vi "Mixing Interface.vi"(10 "Owning VI":refnum<vi>, 11 "Shutdown Event":refnum<user-event>) -> ()   [LabVIEW 2020, in "User Interface.lvlib"]
doc: "Main control interface to Dataflow DJ. Also handles all keyboard shortcuts.\n\n<b>Execution System:</b> User Interface"
uses:
  User Interface.lvlib
  Custom Graphics/Slide.PlaybackPosition.ctl
  Custom Graphics/WaveformGraph.WaveformDisplay.ctl
  Custom Graphics/Button.Large.ctl
  Custom Graphics/LED.Red.16px.ctl
  <vilib>/Utility/miscctls.llb/LVCursorListTypeDef.ctl
  Packed Libraries/Audio Processing.lvlibp/Value Properties.ctl
  Packed Libraries/Messaging.lvlibp/Message Cluster.ctl
  Controls/Keyboard Shortcut.ctl
  Knob Fill.vi
  <vilib>/Utility/Data Type/Get Type Information.vi
  Packed Libraries/Messaging.lvlibp
  user32.dll
  Packed Libraries/Audio Processing.lvlibp
panel:
  in  "Transport.Record":T1
  in  "Mixer.Master":dbl(knob)=1.0 caption="MASTER" scale=0.0..1.0
  out "Mixer.Right.LevelIndicator":u8(slide) scale=0.0..20.0
  out "Mixer.Left.LevelIndicator":u8(slide) scale=0.0..20.0
  in  "Sample Pad.13.Trigger":T1
  in  "Sample Pad.14.Trigger":T1
  in  "Sample Pad.15.Trigger":T1
  in  "Sample Pad.16.Trigger":T1
  in  "Sample Pad.9.Trigger":T1
  in  "Sample Pad.10.Trigger":T1
  in  "Sample Pad.11.Trigger":T1
  in  "Sample Pad.12.Trigger":T1
  in  "Sample Pad.5.Trigger":T1
  in  "Sample Pad.6.Trigger":T1
  in  "Sample Pad.7.Trigger":T1
  in  "Sample Pad.8.Trigger":T1
  in  "Sample Pad.4.Trigger":T1
  in  "Sample Pad.3.Trigger":T1
  in  "Sample Pad.2.Trigger":T1
  in  "Sample Pad.1.Trigger":T1
  in  "Transport.Play":T1
  in  "Deck8.PlaybackPosition":T2 scale=0.0..15965568.0
  out "Deck8.Waveform":T3
  out "Deck8.Title":string
  in  "Channel8.Level":dbl(slide)=1.0 scale=0.0..1.0
  in  "EffectUnit8.Effect1.Enable":T4
  out "Channel8.LevelIndicator":u8(slide) scale=0.0..20.0
  in  "EffectUnit8.Effect1":u16(ring)=2 items=["CRUSHER", "ECHO", "FLANGER"]
  in  "Channel8.Gain":dbl(knob)=1.0 caption="GAIN" scale=0.0..2.0
  in  "Channel8.EQFilter":dbl(knob) caption="FILTER" scale=-1.025..1.025
  in  "EffectUnit8.Effect1.Value1":dbl(knob) caption="AMOUNT" scale=0.0..1.0
  in  "EffectUnit8.Effect1.Value2":dbl(knob) caption="SPEED" scale=0.0..0.1
  in  "Deck8.Reverse":T1
  in  "Deck8.Brake":T1
  in  "Deck8.Play":T1
  in  "Deck7.PlaybackPosition":T2 scale=0.0..15965568.0
  out "Deck7.Waveform":T3
  out "Deck7.Title":string
  in  "Channel7.Level":dbl(slide)=1.0 scale=0.0..1.0
  in  "EffectUnit7.Effect1.Enable":T4
  out "Channel7.LevelIndicator":u8(slide) scale=0.0..20.0
  in  "EffectUnit7.Effect1":u16(ring)=2 items=["CRUSHER", "ECHO", "FLANGER"]
  in  "Channel7.Gain":dbl(knob)=1.0 caption="GAIN" scale=0.0..2.0
  in  "Channel7.EQFilter":dbl(knob) caption="FILTER" scale=-1.025..1.025
  in  "EffectUnit7.Effect1.Value1":dbl(knob) caption="AMOUNT" scale=0.0..1.0
  in  "EffectUnit7.Effect1.Value2":dbl(knob) caption="SPEED" scale=0.0..0.1
  in  "Deck7.Reverse":T1
  in  "Deck7.Brake":T1
  in  "Deck7.Play":T1
  in  "Deck6.PlaybackPosition":T2 scale=0.0..15965568.0
  out "Deck6.Waveform":T3
  out "Deck6.Title":string
  in  "Channel6.Level":dbl(slide)=1.0 scale=0.0..1.0
  in  "EffectUnit6.Effect1.Enable":T4
  out "Channel6.LevelIndicator":u8(slide) scale=0.0..20.0
  in  "EffectUnit6.Effect1":u16(ring)=2 items=["CRUSHER", "ECHO", "FLANGER"]
  in  "Channel6.Gain":dbl(knob)=1.0 caption="GAIN" scale=0.0..2.0
  in  "Channel6.EQFilter":dbl(knob) caption="FILTER" scale=-1.025..1.025
  in  "EffectUnit6.Effect1.Value1":dbl(knob) caption="AMOUNT" scale=0.0..1.0
  in  "EffectUnit6.Effect1.Value2":dbl(knob) caption="SPEED" scale=0.0..0.1
  in  "Deck6.Reverse":T1
  in  "Deck6.Brake":T1
  in  "Deck6.Play":T1
  in  "Deck5.PlaybackPosition":T2 scale=0.0..15965568.0
  out "Deck5.Waveform":T3
  out "Deck5.Title":string
  in  "Channel5.Level":dbl(slide)=1.0 scale=0.0..1.0
  in  "EffectUnit5.Effect1.Enable":T4
  out "Channel5.LevelIndicator":u8(slide) scale=0.0..20.0
  in  "EffectUnit5.Effect1":u16(ring)=2 items=["CRUSHER", "ECHO", "FLANGER"]
  in  "Channel5.Gain":dbl(knob)=1.0 caption="GAIN" scale=0.0..2.0
  in  "Channel5.EQFilter":dbl(knob) caption="FILTER" scale=-1.025..1.025
  in  "EffectUnit5.Effect1.Value1":dbl(knob) caption="AMOUNT" scale=0.0..1.0
  in  "EffectUnit5.Effect1.Value2":dbl(knob) caption="SPEED" scale=0.0..0.1
  in  "Deck5.Reverse":T1
  in  "Deck5.Brake":T1
  in  "Deck5.Play":T1
  in  "Deck4.PlaybackPosition":T2 scale=0.0..15965568.0
  out "Deck4.Waveform":T3
  out "Deck4.Title":string
  in  "Channel4.Level":dbl(slide)=1.0 scale=0.0..1.0
  in  "EffectUnit4.Effect1.Enable":T4
  out "Channel4.LevelIndicator":u8(slide) scale=0.0..20.0
  in  "EffectUnit4.Effect1":u16(ring)=2 items=["CRUSHER", "ECHO", "FLANGER"]
  in  "Channel4.Gain":dbl(knob)=1.0 caption="GAIN" scale=0.0..2.0
  in  "Channel4.EQFilter":dbl(knob) caption="FILTER" scale=-1.025..1.025
  in  "EffectUnit4.Effect1.Value1":dbl(knob) caption="AMOUNT" scale=0.0..1.0
  in  "EffectUnit4.Effect1.Value2":dbl(knob) caption="SPEED" scale=0.0..0.1
  in  "Deck4.Reverse":T1
  in  "Deck4.Brake":T1
  in  "Deck4.Play":T1
  in  "Deck3.PlaybackPosition":T2 scale=0.0..10065024.0
  out "Deck3.Waveform":T3
  out "Deck3.Title":string
  in  "Channel3.Level":dbl(slide)=1.0 scale=0.0..1.0
  in  "EffectUnit3.Effect1.Enable":T4
  out "Channel3.LevelIndicator":u8(slide) scale=0.0..20.0
  in  "EffectUnit3.Effect1":u16(ring)=2 items=["CRUSHER", "ECHO", "FLANGER"]
  in  "Channel3.Gain":dbl(knob)=1.0 caption="GAIN" scale=0.0..2.0
  in  "Channel3.EQFilter":dbl(knob) caption="FILTER" scale=-1.025..1.025
  in  "EffectUnit3.Effect1.Value1":dbl(knob) caption="AMOUNT" scale=0.0..1.0
  in  "EffectUnit3.Effect1.Value2":dbl(knob) caption="SPEED" scale=0.0..0.1
  in  "Deck3.Reverse":T1
  in  "Deck3.Brake":T1
  in  "Deck3.Play":T1
  in  "Deck2.PlaybackPosition":T2 scale=0.0..15848064.0
  out "Deck2.Waveform":T3
  out "Deck2.Title":string
  in  "Channel2.Level":dbl(slide)=1.0 scale=0.0..1.0
  in  "EffectUnit2.Effect1.Enable":T4
  out "Channel2.LevelIndicator":u8(slide) scale=0.0..20.0
  in  "EffectUnit2.Effect1":u16(ring)=2 items=["CRUSHER", "ECHO", "FLANGER"]
  in  "Channel2.Gain":dbl(knob)=1.0 caption="GAIN" scale=0.0..2.0
  in  "Channel2.EQFilter":dbl(knob) caption="FILTER" scale=-1.025..1.025
  in  "EffectUnit2.Effect1.Value1":dbl(knob) caption="AMOUNT" scale=0.0..1.0
  in  "EffectUnit2.Effect1.Value2":dbl(knob) caption="SPEED" scale=0.0..0.1
  in  "Deck2.Reverse":T1
  in  "Deck2.Brake":T1
  in  "Deck2.Play":T1
  in  "Deck1.Brake":T1
  in  "Deck1.Reverse":T1
  in  "EffectUnit1.Effect1.Value2":dbl(knob) caption="SPEED" scale=0.0..0.1
  in  "EffectUnit1.Effect1.Value1":dbl(knob) caption="AMOUNT" scale=0.0..1.0
  in  "Channel1.EQFilter":dbl(knob) caption="FILTER" scale=-1.025..1.025
  in  "Channel1.Gain":dbl(knob)=1.0 caption="GAIN" scale=0.0..2.0
  out "Default Value Map":variant=variant("Channel1.EQFilter"=variant(dbl 0.0), "Channel1.EQHigh"=variant(dbl 1.0), "Channel1.EQLow"=variant(dbl 1.0), "Channel1.EQMid"=variant(dbl 1.0), "Channel1.Gain"=variant(dbl 1.0), "Channel1.Level"=variant(dbl 1.0), "Channel2.EQFilter"=variant(dbl 0.0), "Channel2.EQHigh"=variant(dbl 1.0), "Channel2.EQLow"=variant(dbl 1.0), "Channel2.EQMid"=variant(dbl 1.0), "Channel2.Gain"=variant(dbl 1.0), "Channel2.Level"=variant(dbl 1.0), "Deck1.Pitch"=variant(dbl 0.0), "Deck2.Pitch"=variant(dbl 0.0), "EffectUnit1.Effect1.Value1"=variant(dbl 0.0), "EffectUnit1.Effect1.Value2"=variant(dbl 0.0), "EffectUnit1.Effect2.Value1"=variant(dbl 1.0), "EffectUnit1.Effect2.Value2"=variant(dbl 16.0), "EffectUnit1.Effect3.Value1"=variant(dbl 0.0), "EffectUnit1.Effect3.Value2"=variant(dbl 0.0), "EffectUnit2.Effect1.Value1"=variant(dbl 0.0), "EffectUnit2.Effect1.Value2"=variant(dbl 0.0), "EffectUnit2.Effect2.Value1"=variant(dbl 1.0), "EffectUnit2.Effect2.Value2"=variant(dbl 16.0), "EffectUnit2.Effect3.Value1"=variant(dbl 0.0), "EffectUnit2.Effect3.Value2"=variant(dbl 0.0), "Mixer.Crossfader"=variant(dbl 0.0), "Mixer.Headphones"=variant(dbl 1.0), "Mixer.Master"=variant(dbl 1.0))
  in  "EffectUnit1.Effect1.Enable":T4
  in  "EffectUnit1.Effect1":u16(ring)=2 items=["CRUSHER", "ECHO", "FLANGER"]
  out "Channel1.LevelIndicator":u8(slide) scale=0.0..20.0
  in  "Deck1.Play":T1
  out "Deck1.Title":string
  in  "Channel1.Level":dbl(slide)=1.0 scale=0.0..1.0
  in  "Deck1.PlaybackPosition":T2 scale=0.0..7459200.0
  out "Deck1.Waveform":T3
  # "TRANSPORT"
  # "SAMPLE PAD"
  # "CHANNEL 1"
  # "CHANNEL 2"
  # "CHANNEL 3"
  # "CHANNEL 4"
  # "CHANNEL 5"
  # "CHANNEL 6"
  # "CHANNEL 7"
  # "CHANNEL 8"
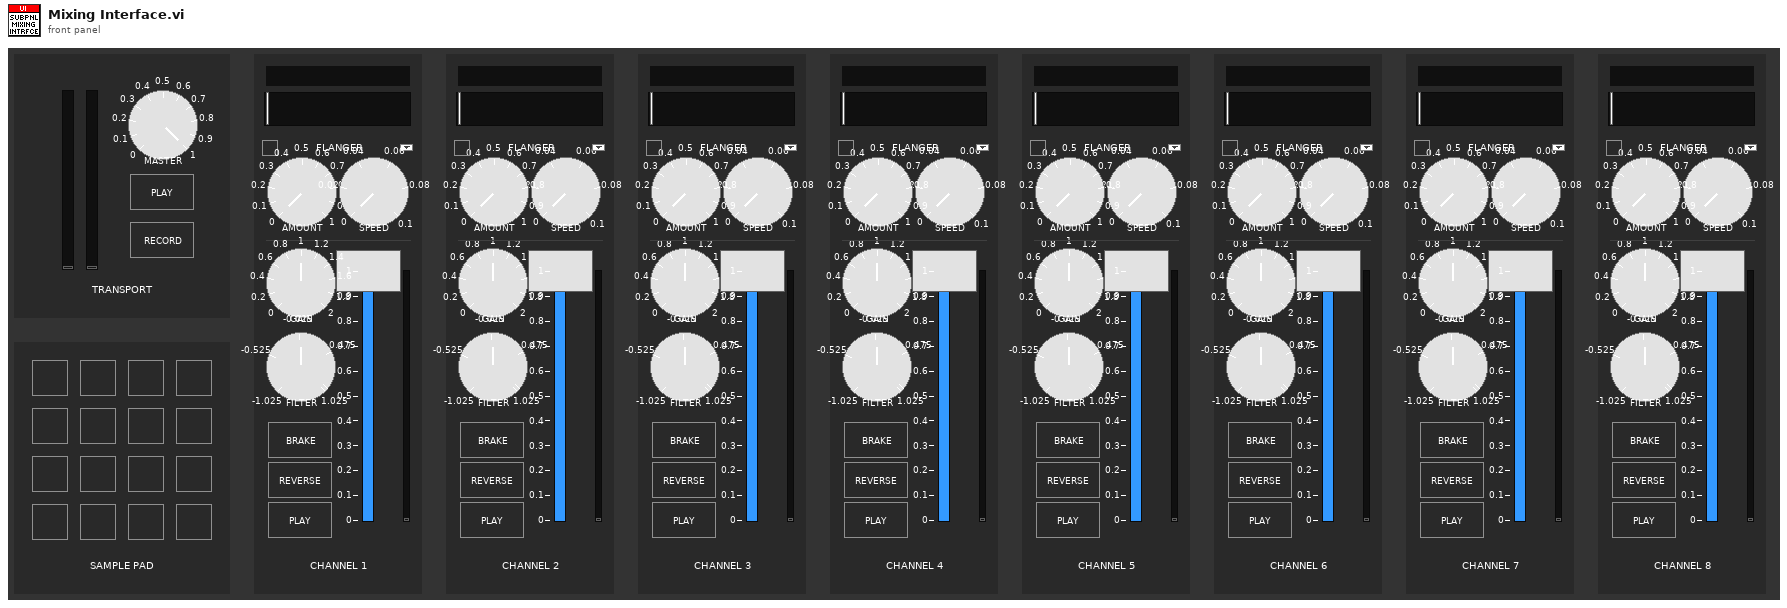
[diagram p1: front panel]
types:
  T1 = typedef "User Interface.lvlib/Button.Large.ctl" = bool
  T2 = typedef "User Interface.lvlib/Slide.PlaybackPosition.ctl" = i32
  T3 = typedef "User Interface.lvlib/WaveformGraph.WaveformDisplay.ctl" = dbl[][]
  T4 = typedef "User Interface.lvlib/LED.Red.16px.ctl" = bool
  T5 = typedef "LVCursorListTypeDef.ctl" = cluster{"Name":string, "Color":u32, "Style":u8, "Point Style":u8, "Name Visible":bool, "Allow Drag":bool, "Cursor Mode":u32, "Plot":i32, "Index":i32, "Position":cluster{"X":dbl, "Y":dbl}, "X Scale":u32, "Y Scale":u32, "Watch Plots":i32[], "Watch All Plots":bool, "Plot Area":i32, "Label Offset":cluster{"X":dbl, "Y":dbl}}[]
  T6 = typedef "Keyboard Shortcut.ctl" = cluster{"Keystroke":string, "Message Queue":string, "Event":string, "Target":string, "Data":variant}
  T7 = typedef "Audio Processing.lvlibp/Value Properties.ctl" = cluster{"Lower":dbl, "Upper":dbl, "Default":dbl, "Increment":dbl}
  T8 = typedef "Messaging.lvlib/Message Cluster.ctl" = cluster{"Event":string, "Source":string, "Target":string, "Data":variant}
  T9 = typedef "Messaging.lvlibp/Message Cluster.ctl" = cluster{"Event":string, "Source":string, "Target":string, "Data":variant}
  T10 = cluster{"type":i32, "KEYBDINPUT":cluster{"dx":i32, "dy":i32, "mouseData":i32, "dwFlags":i32, "time":i32, "dwExtraInfo":u32}}
  T11 = typedef "eventvkey.ctl" = enum16{"ASCII", "Enter", "Return", "Shift", "Ctrl", "Alt", "Cmd", "Opt", "Caps", "NumLock", "Clear", "Break", "Up", "Down", "Left", "Right", "Insert", "Delete", "Home", "End", "PageUp", "PageDown", "Escape", "Help", "Pause", "ScrollLock", "F1", "F2", "F3", "F4", "F5", "F6", "F7", "F8", "F9", "F10", "F11", "F12", "F13", "F14", "F15", "F16", "F17", "F18", "F19", "F20", "F21", "F22", "F23", "F24", "Play", "VolumeUp", "VolumeDown", "Mute", "Two Byte Char"}
  T12 = cluster{"Shift":bool, "Ctrl":bool, "Alt":bool, "Cmd":bool, "Opt":bool}
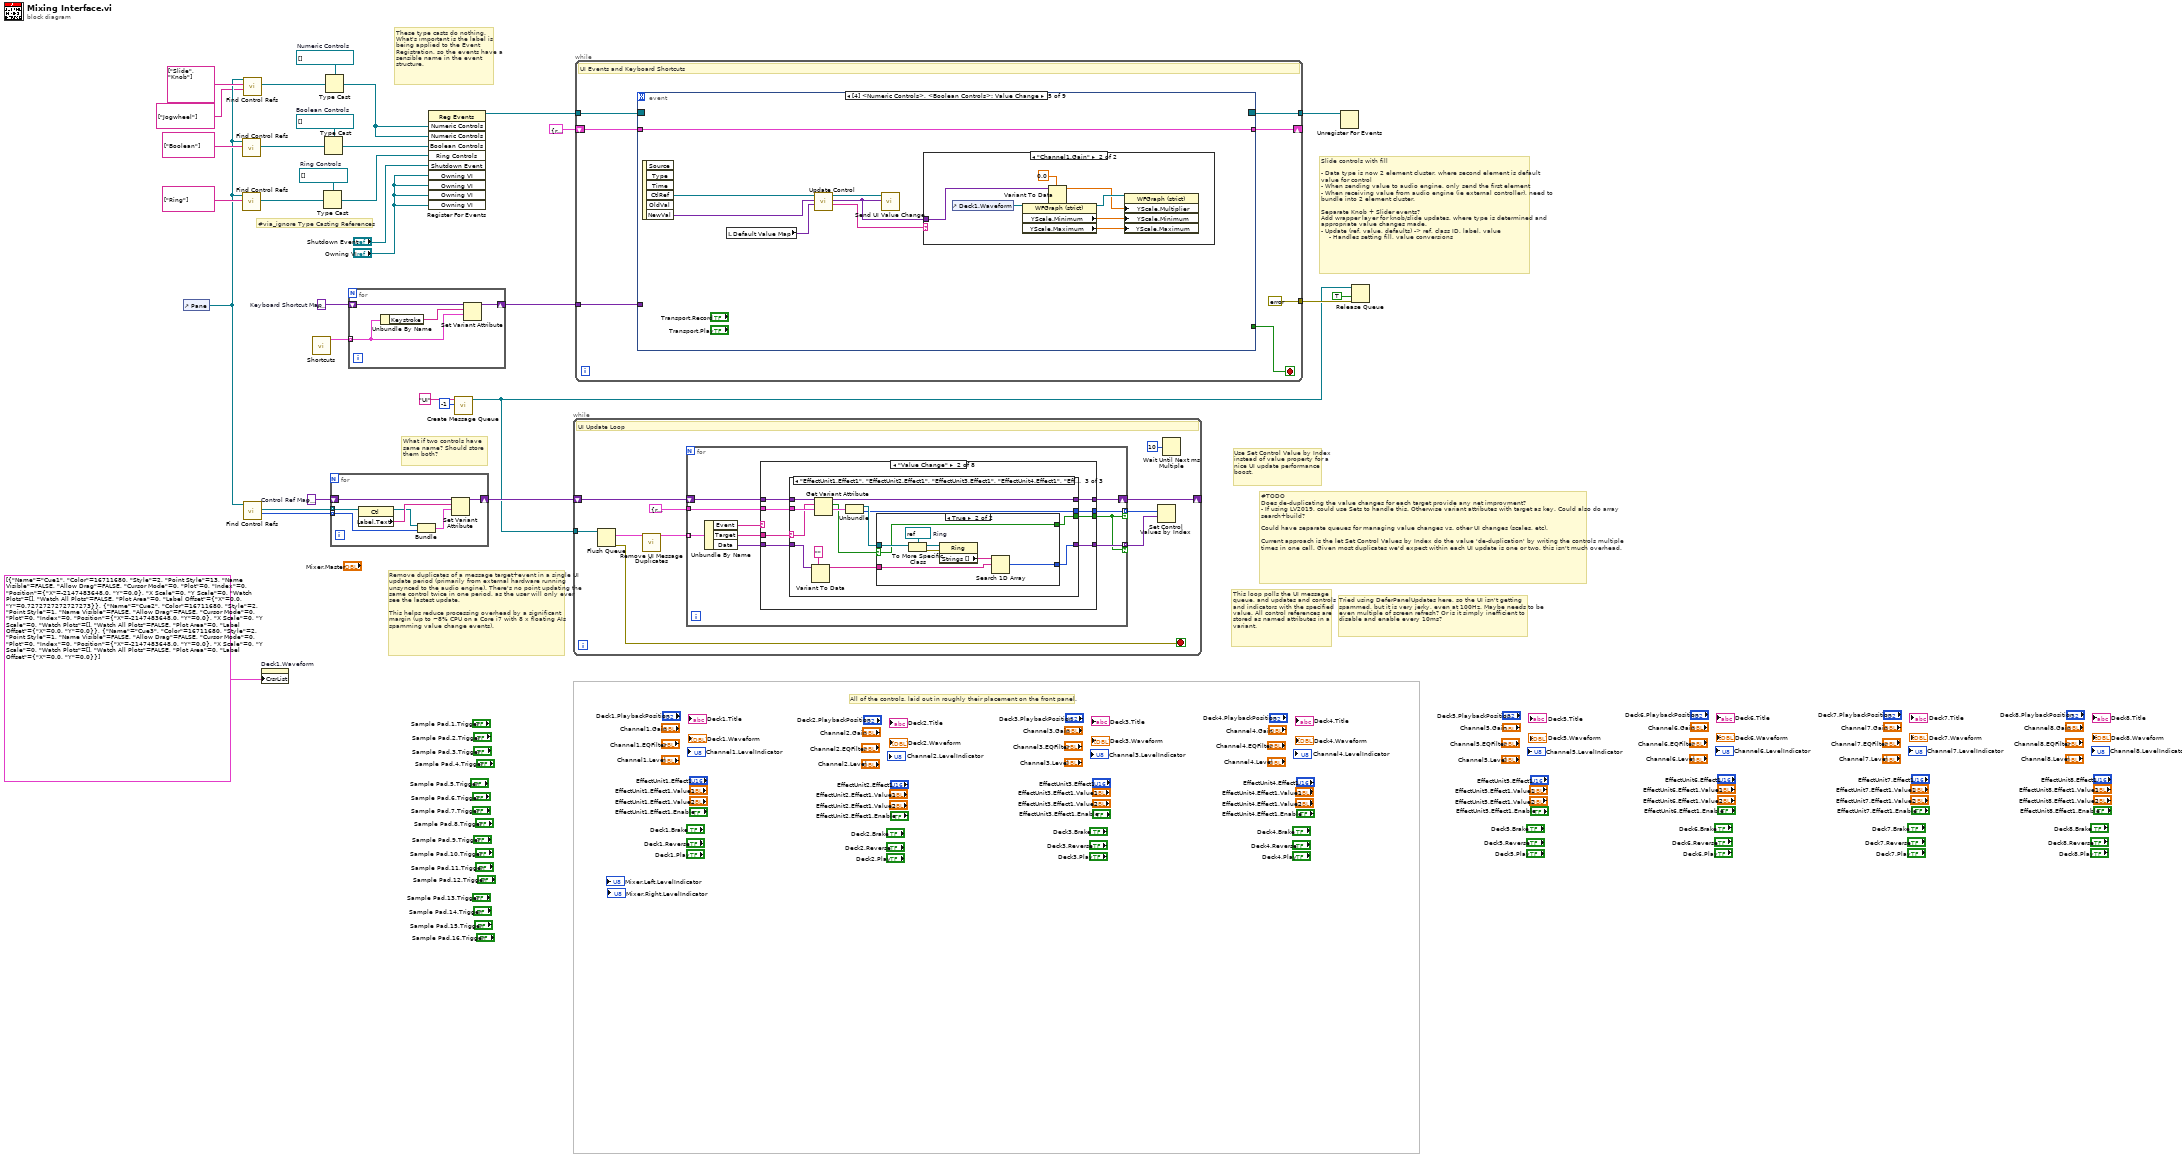
[diagram p0: block diagram]
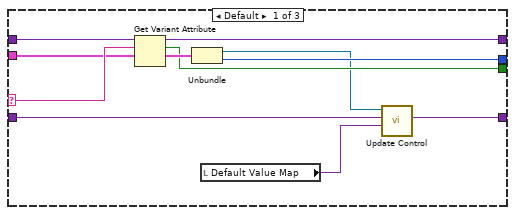
[diagram p3: hidden frame]
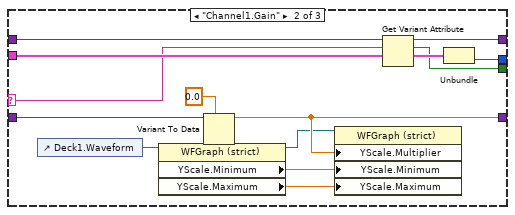
[diagram p4: hidden frame]
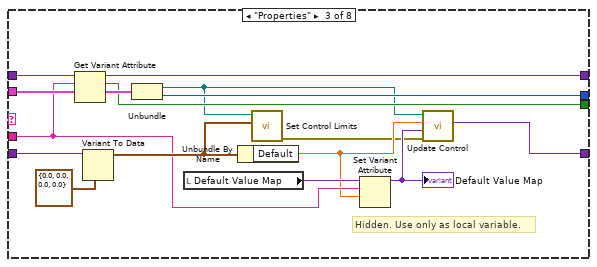
[diagram p6: hidden frame]
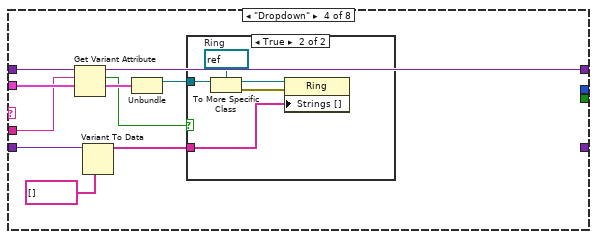
[diagram p7: hidden frame]
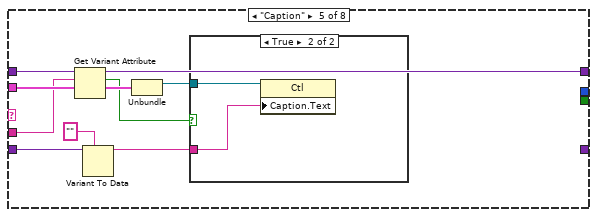
[diagram p9: hidden frame]
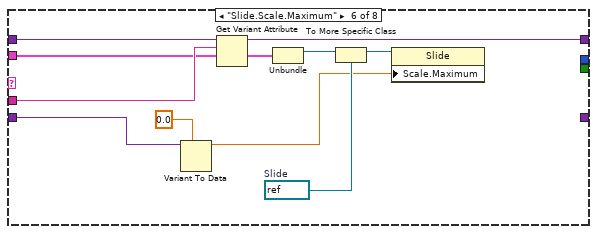
[diagram p11: hidden frame]
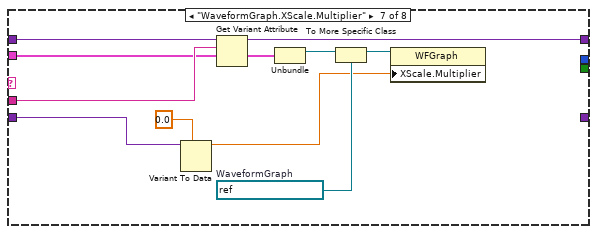
[diagram p12: hidden frame]
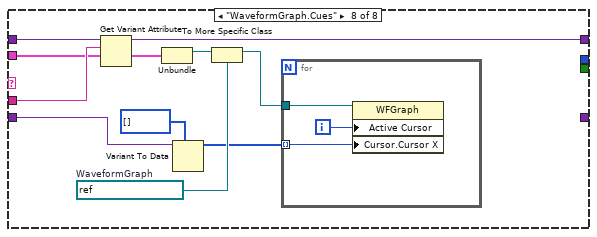
[diagram p13: hidden frame]
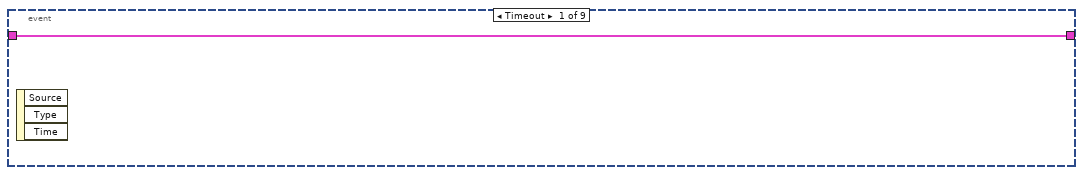
[diagram p14: hidden frame]
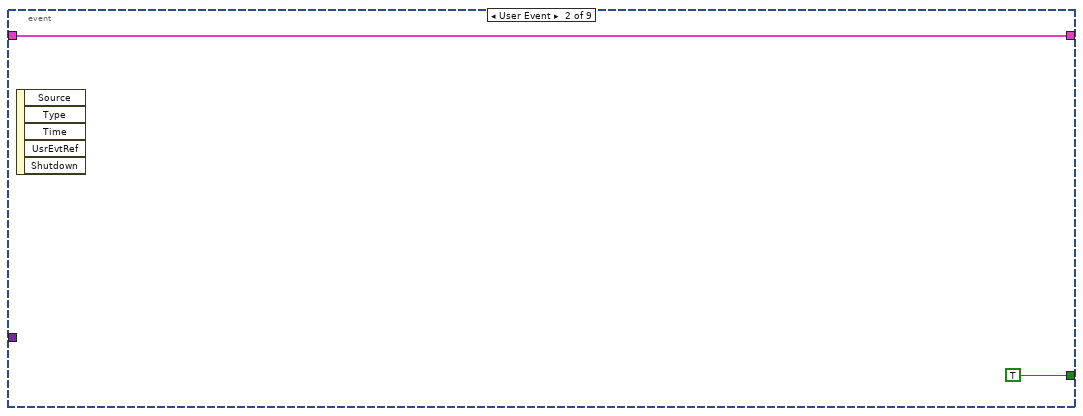
[diagram p15: hidden frame]
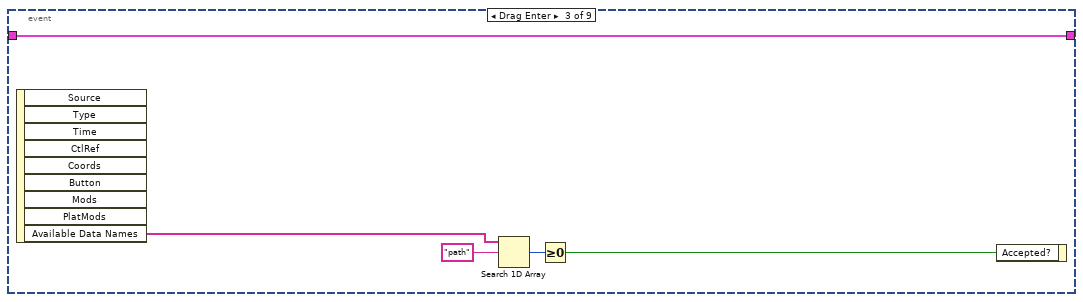
[diagram p16: hidden frame]
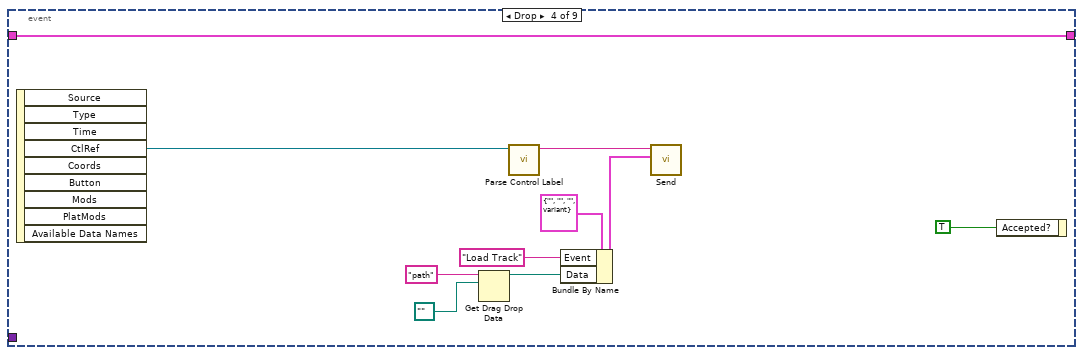
[diagram p17: hidden frame]
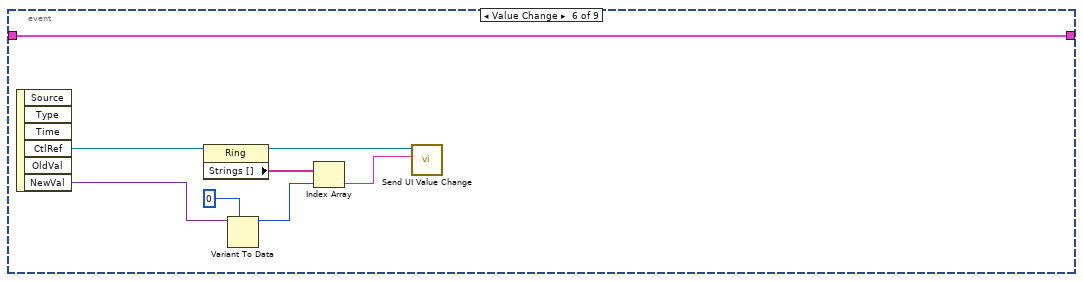
[diagram p19: hidden frame]
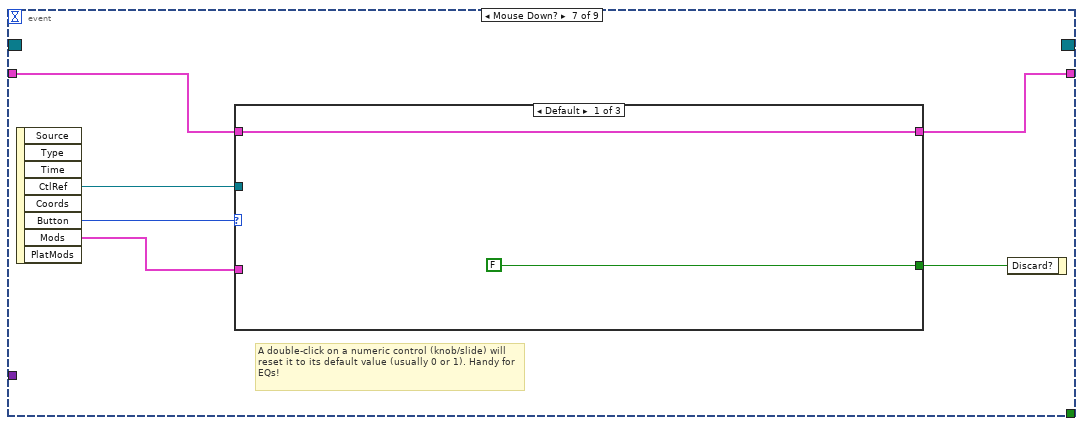
[diagram p20: hidden frame]
diagram:
  w6 = refnum<vi>[] []  # Ring Controls
  w24 = variant  # Keyboard Shortcut Map
  w27 = variant  # Control Ref Map
  w31 = refnum<vi>[] []  # Boolean Controls
  w30 = refnum<vi>[] []  # Numeric Controls
  # "Remove duplicates of a message target+event in a single UI update period (primarily from external hardware running unsynced to the audio engine). There's no point updating the same control twice in one period, as the user will only ever see the lastest update.\n\nThis helps reduce processing overhead by a significant margin (up to ~8% CPU on a Core i7 with 8 x floating AIs spamming value change events)."
  # "Slide controls with fill\n\n- Data type is now 2 element cluster, where second element is default value for control\n- When sending value to audio engine, only send the first element\n- When receiving value from audio engine (ie external controller), need to bundle into 2 element cluster.\n\nSeparate Knob + Slider events?\nAdd wrapper layer for knob/slide updates, where type is determined and appropriate value changes made.\n- Update (ref, value, defaults) -> ref, class ID, label, value\n    - Handles setting fill, value conversions"
  # "#via_ignore Type Casting References"
  # "Use Set Control Value by Index instead of value property for a nice UI update performance boost."
  # "#TODO\nDoes de-duplicating the value changes for each target provide any net improvment?\n- If using LV2019, could use Sets to handle this. Otherwise variant attributes with target as key. Could also do array search+build?\n\nCould have separate queues for managing value changes vs. other UI changes (scales, etc).\n\nCurrent approach is the let Set Control Values by Index do the value 'de-duplication' by writing the controls multiple times in one call. Given most duplicates we'd expect within each UI update is one or two, this isn't much overhead."
  # "What if two controls have same name? Should store them both?"
  # "All of the controls, laid out in roughly their placement on the front panel."
  # "This loop polls the UI message queue, and updates and controls and indicators with the specified value. All control references are stored as named attributes in a variant."
  # "Tried using DeferPanelUpdates here, so the UI isn't getting spammed, but it is very jerky, even at 100Hz. Maybe needs to be even multiple of screen refresh? Or is it simply inefficient to disable and enable every 10ms?"
  # "These type casts do nothing. What's important is the label is being applied to the Event Registration, so the events have a sensible name in the event structure."
  n1 = control-ref of="Pane"() -> (w2:refnum<vi>)
  n2 = call "Find Control Refs.vi"("Control Types"=string[] ["Boolean"], "Pane Reference In"=w2) -> ("Control Refs"=w15:refnum<vi>[])  [unwired: 7 in, 2 out]
  n3 = call "Find Control Refs.vi"("Control Types"=string[] ["Ring"], "Pane Reference In"=w2) -> ("Control Refs"=w5:refnum<vi>[])  [unwired: 7 in, 2 out]
  n4 = call "Find Control Refs.vi"("Pane Reference In"=w2) -> ("Control Indicies"=w8:i32[], "Control Refs"=w14:refnum<vi>[])  [unwired: 8 in, 1 out]
  n5 = call "Find Control Refs.vi"("Label.Text Filter"=string[] ["Jogwheel"], "Control Types"=string[] ["Slide", "Knob"], "Pane Reference In"=w2) -> ("Control Refs"=w9:refnum<vi>[])  [unwired: 6 in, 2 out]
  n6 = property on="Deck1.Waveform" class="WFGraph (strict)"("CrsrList"=T5 [{"Name"="Cue1", "Color"=16711680, "Style"=2, "Point Style"=13, "Name Visible"=FALSE, "Allow Drag"=FALSE, "Cursor Mode"=0, "Plot"=0, "Index"=0, "Position"={"X"=-2147483648.0, "Y"=0.0}, "X Scale"=0, "Y Scale"=0, "Watch Plots"=[], "Watch All Plots"=FALSE, "Plot Area"=0, "Label Offset"={"X"=0.0, "Y"=0.7272727272727273}}, {"Name"="Cue2", "Color"=16711680, "Style"=2, "Point Style"=1, "Name Visible"=FALSE, "Allow Drag"=FALSE, "Cursor Mode"=0, "Plot"=0, "Index"=0, "Position"={"X"=-2147483648.0, "Y"=0.0}, "X Scale"=0, "Y Scale"=0, "Watch Plots"=[], "Watch All Plots"=FALSE, "Plot Area"=0, "Label Offset"={"X"=0.0, "Y"=0.0}}, {"Name"="Cue3", "Color"=16711680, "Style"=2, "Point Style"=1, "Name Visible"=FALSE, "Allow Drag"=FALSE, "Cursor Mode"=0, "Plot"=0, "Index"=0, "Position"={"X"=-2147483648.0, "Y"=0.0}, "X Scale"=0, "Y Scale"=0, "Watch Plots"=[], "Watch All Plots"=FALSE, "Plot Area"=0, "Label Offset"={"X"=0.0, "Y"=0.0}}] ("Cursor List")) -> ()  [unwired: 2 in, 2 out]
  n7 = call "Shortcuts.vi"() -> ("Keyboard Shortcuts"=w22:T6[])  [unwired: 11 in]
  n8 = Type Cast(type=w6, x=w5) -> (*(type *) &x=w4:refnum<vi>[])
  n9 = Type Cast(type=w31, x=w15) -> (*(type *) &x=w28:refnum<vi>[])
  n10 = Type Cast(type=w30, x=w9) -> (*(type *) &x=w13:refnum<vi>[])
  n11 = for {
    shift-right: [w38] -> w26
    shift-left: w27 -> [w39]
    tunnel: w14 -> [w37] mode=indexing
    tunnel: w8 -> [w34] mode=indexing
    n12 = property class="Ctl"(reference=w37) -> (reference out=w35:refnum<vi>, "Label.Text"=w36:string)  [unwired: 1 in, 1 out]
    n13 = Bundle(w35, w34) -> (w33:cluster{refnum<vi>, i32})  [unwired: 1 in]
    n14 = Set Variant Attribute(Variant=w39, name=w36, value=w33) -> (Variant out=w38:variant)  [unwired: 1 in, 2 out]
  }
  n15 = for {
    shift-right: [w42] -> w23
    shift-left: w24 -> [w43]
    tunnel: w22 -> [w40] mode=indexing
    n16 = Unbundle By Name(w40) -> ("Keystroke"=w41:string)
    n17 = Set Variant Attribute(Variant=w43, name=w41, value=w40) -> (Variant out=w42:variant)  [unwired: 1 in, 2 out]
  }
  n18 = register-events(w13, w13, w28, w4, "Shutdown Event", "Owning VI", "Owning VI", "Owning VI", "Owning VI") -> (reference out=w32:refnum<event-registration>)  [unwired: 2 in, 1 out]
  n19 = call "Create Message Queue.vi"("Max Size (1000)"=-1, "Queue Name"="UI") -> ("queue out"=w18:refnum<queue>)  [unwired: 8 in, 1 out]
  n20 = while {
    tunnel: w18 -> [w51]
    shift-right: [w52] -> _
    shift-left: w26 -> [w53]
    stop <- w49 stop-if-true
    # "UI Update Loop"
    n21 = Flush Queue(queue=w51) -> (remaining elements=w45:T8[], error out=w49:errorcluster)  [unwired: 1 in, 1 out]
    n22 = call "Remove UI Message Duplicates.vi"("Messages In"=w45) -> ("Messages Out"=w44:T9[])  [unwired: 10 in]
    n23 = for {
      shift-right: [w62] -> w52
      shift-left: w53 -> [w63]
      tunnel: w44 -> [w58] mode=indexing
      tunnel: cluster{refnum<vi>, i32} {refnum, 0} ("output cluster") -> [w57]
      tunnel: [w56] -> w47 mode=indexing if=w54
      tunnel: [w55] -> w46 mode=indexing if=w54
      n24 = Unbundle By Name(w58) -> ("Event"=w61:string, "Target"=w59:string, "Data"=w60:variant)
      n25 = case shown="\"Value Change\"" w61 {
        tunnel: w63 -> [w65 w73 w133 w144 w158 w174 w185 w196]
        tunnel: w59 -> [_ w70 w126 w141 w155 w172 w183 w194]
        tunnel: [w65 w72 w132 w143 w157 w173 w184 w195] -> w62
        tunnel: w60 -> [w64 w71 w135 w146 w160 w168 w179 w190]
        tunnel: w57 -> [_ w69 w130 w142 w156 w166 w177 w188]
        tunnel: [_ w68 w131 _ _ _ _ _] -> w56
        tunnel: [_ w66 w129 _ _ _ _ _] -> w54
        tunnel: [w64 w67 w122 _ _ _ _ _] -> w55
        frame Default {
        }
        frame "Value Change" {
          n26 = case shown="\"EffectUnit1.Effect1\", \"EffectUnit2.Effect1\", \"EffectUnit3.Effect1\", \"EffectUnit4.Effect1\", \"EffectUnit5.Effect1\", \"EffectUnit6.Effect1\", \"EffectUnit7.Effect1\", \"EffectUnit8.Effect1\"" w70 {
            selector: w70 -> [w82 w89 w108]
            tunnel: w73 -> [w84 w98 w110]
            tunnel: [w83 w97 w107] -> w72
            tunnel: w71 -> [w76 w91 w104]
            tunnel: w69 -> [w81 w95 w109]
            tunnel: [w79 w93 w100] -> w68
            tunnel: [w75 w86 w101] -> w67
            tunnel: [w78 w92 w99] -> w66
            frame Default {
              n27 = Get Variant Attribute(Variant=w84, name=w82, default value (empty Variant)=w81) -> (duplicate Variant=w83:variant, found=w78:bool, value=w80:cluster{refnum<vi>, i32})  [unwired: 1 in, 1 out]
              n28 = Unbundle(w80) -> (w77:refnum<vi>, w79:i32)
              n29 = local read "Default Value Map"() -> (w74:variant)
              n30 = call "Update Control.vi"("Default Value Map"=w74, "Value In"=w76, "Control Ref"=w77) -> ("Value Out"=w75:variant)  [unwired: 5 in, 3 out]
            }
            frame "Channel1.Gain" {
              n31 = control-ref of="Deck1.Waveform"() -> (w90:refnum<vi>)
              n32 = property class="WFGraph (strict)"(reference=w90) -> (reference out=w85:refnum<vi>, "YScale.Minimum"=w88:dbl, "YScale.Maximum"=w87:dbl)  [unwired: 1 in, 1 out]
              n33 = Variant To Data(type=0.0 ("y"), Variant=w91) -> (data=w86:dbl)  [unwired: 1 in, 1 out]
              n34 = property class="WFGraph (strict)"(reference=w85, "YScale.Multiplier"=w86, "YScale.Minimum"=w88, "YScale.Maximum"=w87) -> ()  [unwired: 1 in, 2 out]
              n35 = Get Variant Attribute(Variant=w98, name=w89, default value (empty Variant)=w95) -> (duplicate Variant=w97:variant, found=w92:bool, value=w94:cluster{refnum<vi>, i32})  [unwired: 1 in, 1 out]
              n36 = Unbundle(w94) -> (w93:i32)  [unwired: 1 out]
            }
            frame "EffectUnit1.Effect1", "EffectUnit2.Effect1", "EffectUnit3.Effect1", "EffectUnit4.Effect1", "EffectUnit5.Effect1", "EffectUnit6.Effect1", "EffectUnit7.Effect1", "EffectUnit8.Effect1" {
              n37 = Variant To Data(type="", Variant=w104) -> (data=w102:string)  [unwired: 1 in, 1 out]
              n38 = Get Variant Attribute(Variant=w110, name=w108, default value (empty Variant)=w109) -> (duplicate Variant=w107:variant, found=w106:bool, value=w111:cluster{refnum<vi>, i32})  [unwired: 1 in, 1 out]
              n39 = Unbundle(w111) -> (w105:refnum<vi>, w100:i32)
              n40 = case shown="True" w106 {
                selector: w106 -> [w112 w113]
                tunnel: w105 -> [_ w120]
                tunnel: w102 -> [_ w116]
                tunnel: [_ w114] -> w101
                tunnel: [w112 w113] -> w99
                frame False {
                }
                frame True {
                  w119 = refnum<vi> refnum  # Ring
                  n41 = To More Specific Class(target class=w119, reference=w120) -> (specific class reference=w118:refnum<vi>, error out=w115:errorcluster)  [unwired: 1 in]
                  n42 = property class="Ring"(reference=w118, error in=w115) -> ("Strings []"=w117:string[])  [unwired: 2 out]
                  n43 = Search 1D Array(1D array=w117, element=w116) -> (index of element=w114:i32)  [unwired: 1 in]
                }
              }
            }
          }
        }
        frame "Properties" {
          # "Hidden. Use only as local variable."
          n44 = Get Variant Attribute(Variant=w133, name=w126, default value (empty Variant)=w130) -> (duplicate Variant=w132:variant, found=w129:bool, value=w134:cluster{refnum<vi>, i32})  [unwired: 1 in, 1 out]
          n45 = Variant To Data(type=T7 {"Lower"=0.0, "Upper"=0.0, "Default"=0.0, "Increment"=0.0} ("Value Properties"), Variant=w135) -> (data=w128:T7)  [unwired: 1 in, 1 out]
          n46 = Unbundle(w134) -> (w125:refnum<vi>, w131:i32)
          n47 = local read "Default Value Map"() -> (w127:variant)
          n48 = Unbundle By Name(w128) -> ("Default"=w124:dbl)
          n49 = call "Set Control Limits.vi"("Value Properties"=w128, "Control Ref"=w125) -> ("error out"=w121:errorcluster)  [unwired: 9 in]
          n50 = Set Variant Attribute(Variant=w127, name=w126, value=w124) -> (Variant out=w123:variant)  [unwired: 1 in, 2 out]
          "Default Value Map" <- w123
          n51 = call "Update Control.vi"("error in (no error)"=w121, "Default Value Map"=w123, "Value In"=w124, "Control Ref"=w125) -> ("Value Out"=w122:variant)  [unwired: 4 in, 3 out]
        }
        frame "Dropdown" {
          n52 = Get Variant Attribute(Variant=w144, name=w141, default value (empty Variant)=w142) -> (duplicate Variant=w143:variant, found=w139:bool, value=w145:cluster{refnum<vi>, i32})  [unwired: 1 in, 1 out]
          n53 = Variant To Data(type=string[] [], Variant=w146) -> (data=w137:string[])  [unwired: 1 in, 1 out]
          n54 = Unbundle(w145) -> (w138:refnum<vi>)  [unwired: 1 out]
          n55 = case shown="True" w139 {
            tunnel: w138 -> [_ w151]
            tunnel: w137 -> [_ w148]
            frame False {
            }
            frame True {
              w149 = refnum<vi> refnum  # Ring
              n56 = To More Specific Class(target class=w149, reference=w151) -> (specific class reference=w150:refnum<vi>, error out=w147:errorcluster)  [unwired: 1 in]
              n57 = property class="Ring"(reference=w150, error in=w147, "Strings []"=w148) -> ()  [unwired: 2 out]
            }
          }
        }
        frame "Caption" {
          n58 = Get Variant Attribute(Variant=w158, name=w155, default value (empty Variant)=w156) -> (duplicate Variant=w157:variant, found=w154:bool, value=w159:cluster{refnum<vi>, i32})  [unwired: 1 in, 1 out]
          n59 = Variant To Data(type="", Variant=w160) -> (data=w152:string)  [unwired: 1 in, 1 out]
          n60 = Unbundle(w159) -> (w153:refnum<vi>)  [unwired: 1 out]
          n61 = case shown="True" w154 {
            tunnel: w153 -> [_ w163]
            tunnel: w152 -> [_ w162]
            frame False {
            }
            frame True {
              n62 = property class="Ctl"(reference=w163, "Caption.Text"=w162) -> ()  [unwired: 1 in, 2 out]
            }
          }
        }
        frame "Slide.Scale.Maximum" {
          w171 = refnum<vi> refnum  # Slide
          n63 = Variant To Data(type=0.0, Variant=w168) -> (data=w169:dbl)  [unwired: 1 in, 1 out]
          n64 = Get Variant Attribute(Variant=w174, name=w172, default value (empty Variant)=w166) -> (duplicate Variant=w173:variant, value=w165:cluster{refnum<vi>, i32})  [unwired: 1 in, 2 out]
          n65 = Unbundle(w165) -> (w164:refnum<vi>)  [unwired: 1 out]
          n66 = To More Specific Class(target class=w171, reference=w164) -> (specific class reference=w170:refnum<vi>)  [unwired: 1 in, 1 out]
          n67 = property class="Slide"(reference=w170, "Scale.Maximum"=w169) -> ()  [unwired: 1 in, 2 out]
        }
        frame "WaveformGraph.XScale.Multiplier" {
          w182 = refnum<vi> refnum  # WaveformGraph
          n68 = Variant To Data(type=0.0, Variant=w179) -> (data=w180:dbl)  [unwired: 1 in, 1 out]
          n69 = Get Variant Attribute(Variant=w185, name=w183, default value (empty Variant)=w177) -> (duplicate Variant=w184:variant, value=w176:cluster{refnum<vi>, i32})  [unwired: 1 in, 2 out]
          n70 = Unbundle(w176) -> (w175:refnum<vi>)  [unwired: 1 out]
          n71 = To More Specific Class(target class=w182, reference=w175) -> (specific class reference=w181:refnum<vi>)  [unwired: 1 in, 1 out]
          n72 = property class="WFGraph"(reference=w181, "XScale.Multiplier"=w180) -> ()  [unwired: 1 in, 2 out]
        }
        frame "WaveformGraph.Cues" {
          w193 = refnum<vi> refnum  # WaveformGraph
          n73 = Get Variant Attribute(Variant=w196, name=w194, default value (empty Variant)=w188) -> (duplicate Variant=w195:variant, value=w187:cluster{refnum<vi>, i32})  [unwired: 1 in, 2 out]
          n74 = Unbundle(w187) -> (w186:refnum<vi>)  [unwired: 1 out]
          n75 = Variant To Data(type=i32[] [], Variant=w190) -> (data=w191:i32[])  [unwired: 1 in, 1 out]
          n76 = To More Specific Class(target class=w193, reference=w186) -> (specific class reference=w192:refnum<vi>)  [unwired: 1 in, 1 out]
          n77 = for {
            tunnel: w192 -> [w199]
            tunnel: w191 -> [w198] mode=indexing
            i -> [w197]
            n78 = property class="WFGraph"(reference=w199, "Active Cursor"=w197, "Cursor.Cursor X"=w198) -> ()  [unwired: 1 in, 2 out]
          }
        }
      }
    }
    n79 = Set Control Values by Index(1:w47, 2:w46) -> ()  [unwired: 2 in, 1 out]
    n80 = Wait Until Next ms Multiple(millisecond multiple=u32 10) -> ()  [unwired: 1 out]
  }
  n81 = while {
    tunnel: [errorcluster {"status"=FALSE, "code"=0, "source"=""} ("error in (no error)")] -> w25
    tunnel: w32 -> [w205]
    tunnel: [w204] -> w29
    tunnel: w23 -> [w203]
    shift-right: [w201] -> _
    shift-left: cluster{"CtlRef":refnum<vi>, "Value":variant} {"CtlRef"=refnum, "Value"=variant} -> [w200]
    stop <- w202 stop-if-true
    # "UI Events and Keyboard Shortcuts"
    n82 = event shown="[4] <Numeric Controls>, <Boolean Controls>: Value Change" {
      selector: w205 -> [_ _ _ _ _ _ _ _ _]
      dyn-events: [_ _ _ _ _ _ _ _ _] -> w204
      timeout: _ -> [_ _ _ _ _ _ _ _ _]
      tunnel: w203 -> [_ _ _ _ _ _ _ w289 _]
      tunnel: [_ TRUE _ _ _ _ _ _ _] -> w202
      tunnel: [w207 w208 w210 w215 w231 w246 w249 w283 w302] -> w201
      tunnel: w200 -> [w207 w208 w210 w215 w231 w246 w248 w283 w303]
      event Timeout {
        n83 = event-data() -> ()  [unwired: 1 in, 3 out]
      }
      event User Event {
        n84 = event-data() -> ()  [unwired: 1 in, 5 out]
      }
      event Drag Enter {
        n85 = event-data() -> ("Available Data Names"=w212:string[])  [unwired: 1 in, 8 out]
        n86 = Search 1D Array(1D array=w212, element="path") -> (index of element=w213:i32)  [unwired: 1 in]
        n87 = Greater Or Equal To 0?(x=w213) -> (x >= 0?=w211:bool)
        n88 = event-data("Accepted?"=w211) -> ()  [unwired: 1 in, 1 out]
      }
      event Drop {
        n89 = event-data() -> ("CtlRef"=w218:refnum<vi>)  [unwired: 1 in, 8 out]
        n90 = Get Drag Drop Data(8:path "", 9:"path" ("data name")) -> (3:w216:path)  [unwired: 1 in, 1 out]
        n91 = call "Parse Control Label.vi"("CtlRef"=w218) -> ("Queue Name"=w217:string)  [unwired: 9 in, 1 out]
        n92 = Bundle By Name(cluster=T9 {"Event"="", "Source"="", "Target"="", "Data"=variant} ("Message"), "Event"="Load Track" ("Type"), "Data"=w216) -> (w220:T9)
        n93 = call "Send.vi"("Message"=w220, "Queue Name"=w217) -> ()  [unwired: 9 in, 1 out]
        n94 = event-data("Accepted?"=TRUE) -> ()  [unwired: 1 in, 1 out]
      }
      event Value Change {
        n95 = event-data() -> ("CtlRef"=w230:refnum<vi>, "NewVal"=w228:variant)  [unwired: 1 in, 4 out]
        n96 = local read "Default Value Map"() -> (w229:variant)
        n97 = call "Update Control.vi"("Default Value Map"=w229, "Value In"=w228, "Control Ref"=w230) -> ("Label Text"=w225:string, "Value Out"=w226:variant, "Control Ref (Dup)"=w227:refnum<vi>)  [unwired: 5 in, 1 out]
        n98 = call "Send UI Value Change.vi"("Data"=w226, "CtlRef"=w227) -> ()  [unwired: 10 in]
        n99 = case shown="\"Channel1.Gain\"" w225 {
          tunnel: w226 -> [_ w233]
          frame Default {
          }
          frame "Channel1.Gain" {
            n100 = control-ref of="Deck1.Waveform"() -> (w237:refnum<vi>)
            n101 = property class="WFGraph (strict)"(reference=w237) -> (reference out=w234:refnum<vi>, "YScale.Minimum"=w236:dbl, "YScale.Maximum"=w235:dbl)  [unwired: 1 in, 1 out]
            n102 = Variant To Data(type=0.0 ("y"), Variant=w233) -> (data=w232:dbl)  [unwired: 1 in, 1 out]
            n103 = property class="WFGraph (strict)"(reference=w234, "YScale.Multiplier"=w232, "YScale.Minimum"=w236, "YScale.Maximum"=w235) -> ()  [unwired: 1 in, 2 out]
          }
        }
      }
      event Value Change {
        n104 = event-data() -> ("CtlRef"=w245:refnum<vi>, "NewVal"=w243:variant)  [unwired: 1 in, 4 out]
        n105 = property class="Ring"(reference=w245) -> (reference out=w244:refnum<vi>, "Strings []"=w241:string[])  [unwired: 1 in, 1 out]
        n106 = Variant To Data(type=u16 0, Variant=w243) -> (data=w240:u16)  [unwired: 1 in, 1 out]
        n107 = Index Array(array=w241, index=w240) -> (element=w239:string)
        n108 = call "Send UI Value Change.vi"("Data"=w239, "CtlRef"=w244) -> ()  [unwired: 10 in]
      }
      event Mouse Down? {
        # "A double-click on a numeric control (knob/slide) will reset it to its default value (usually 0 or 1). Handy for EQs!"
        n109 = event-data() -> ("CtlRef"=w250:refnum<vi>, "Button"=w252:u16, "Mods"=w251:cluster{"Double Click":bool, "Menu Key":bool})  [unwired: 1 in, 5 out]
        n110 = case shown="Default" w252 {
          tunnel: w251 -> [_ w262 _]
          tunnel: w250 -> [_ w258 w278]
          tunnel: [FALSE ("Discard?") w260 TRUE ("Discard?")] -> w247
          tunnel: [w253 w259 w275] -> w249
          tunnel: w248 -> [w253 w259 _]
          frame Default {
          }
          frame 1 {
            n111 = Unbundle By Name(w262) -> ("Double Click"=w261:bool)
            n112 = property class="Ctl"(reference=w258) -> (reference out=w257:refnum<vi>, "Label.Text"=w256:string, "Value"=w255:variant)  [unwired: 1 in, 1 out]
            n113 = case shown="True" w261 {
              tunnel: [FALSE ("Discard?") TRUE ("Discard?")] -> w260
              tunnel: w257 -> [_ w264]
              tunnel: w256 -> [_ w271]
              tunnel: w255 -> [_ w269]
              frame False {
              }
              frame True {
                # "Read and written in Properties case of UI Update Loop."
                n114 = local read "Default Value Map"() -> (w268:variant)
                n115 = Get Variant Attribute(Variant=w268, name=w271, default value (empty Variant)=w269) -> (found=w270:bool, value=w267:variant)  [unwired: 1 in, 2 out]
                n116 = call "Update Control.vi"("Default Value Map"=w268, "Value In"=w267, "Control Ref"=w264) -> ("Value Out"=w266:variant, "Control Ref (Dup)"=w265:refnum<vi>)  [unwired: 5 in, 2 out]
                n117 = case shown="True" w270 {
                  tunnel: w265 -> [_ w274]
                  tunnel: w266 -> [_ w273]
                  frame False {
                  }
                  frame True {
                    n118 = property class="Ctl"(reference=w274, "Val(Sgnl)"=w273) -> ()  [unwired: 1 in, 2 out]
                  }
                }
              }
            }
          }
          frame 2 {
            # "Send a left mouse down"
            n119 = property class="Ctl"(reference=w278) -> (reference out=w277:refnum<vi>, "Value"=w276:variant)  [unwired: 1 in, 1 out]
            n120 = Bundle("CtlRef"=w277, "Value"=w276) -> (w275:cluster{"CtlRef":refnum<vi>, "Value":variant})  [unwired: 1 in]
            n121 = dll-call lib="user32.dll" fn="SendInput"("nInputs"=u32 1, "pInputs"=T10 {"type"=0, "KEYBDINPUT"={"dx"=0, "dy"=0, "mouseData"=0, "dwFlags"=2, "time"=0, "dwExtraInfo"=0}} ("input"), "cbSize"=u32 28) -> ()  [unwired: 7 in, 2 out]
          }
        }
        n122 = event-data("Discard?"=w247) -> ()  [unwired: 1 in, 1 out]
      }
      event Key Down?; event type 5.0.x8000000b; event type 1.0.x8000000b {
        # "Register Key Down events on both THIS VI (running in a sub panel), and the owning VI. Why both? Why not just the owning VI?\n\nUsing just the Key Down event from the owning VI works, EXCEPT for when the mouse is being held down at the same time. LabVIEW seems to redirect all input focus to the sub panel VI (this VI) while the mouse button is being held. As such the owning VI can no longer generate Key Down events."
        # "#BUG\nWhile holding the mouse button down on a control (moving a slider for example), F10 will not register as a key press. All other function keys seem to work.\n\nWTF.\n\nHelp mentions F3 being an issue, but that's always worked. F1 will trigger the LabVIEW help if the key press isn't discarded."
        # "#TODO\nIf file browser controls are in focus, don't execute shortcuts? Or at least allow certain key presses (arrow keys, pgup, pgdwn, home, end, etc)"
        # "Always discard the key press, and don't pass them on to controls or LabVIEW itself."
        # "Keyboard shortcuts can be setup directly on a control, but LabVIEW only supports function keys and other non-ASCII inputs. In this case we want any key to be a possible shortcut, so all key presses are captured here."
        n123 = event-data() -> ("VKey"=w285:T11, "ScanCode"=w286:i16, "Mods"=w287:cluster{"Num Pad":bool, "Menu Key":bool}, "PlatMods"=w288:T12)  [unwired: 1 in, 6 out]
        n124 = call "Parse Key Press.vi"("PlatMods"=w288, "Mods"=w287, "ScanCode"=w286, "VKey"=w285) -> ("Key Pressed"=w290:string)  [unwired: 7 in]
        n125 = Get Variant Attribute(Variant=w289, name=w290, default value (empty Variant)=T6 {"Keystroke"="", "Message Queue"="", "Event"="", "Target"="", "Data"=variant(bool FALSE)}) -> (found=w292:bool, value=w291:T6)  [unwired: 1 in, 2 out]
        n126 = case shown="True" w292 {
          tunnel: w291 -> [_ w301]
          frame False {
          }
          frame True {
            n127 = Unbundle By Name(w301) -> ("Message Queue"=w300:string, "Event"=w297:string, "Target"=w296:string, "Data"=w294:variant)
            n128 = Bundle By Name(cluster=T9 {"Event"="", "Source"="", "Target"="", "Data"=variant} ("Message"), "Event"=w297, "Target"=w296, "Data"=w294, "Source"="Shortcut") -> (w298:T9)
            n129 = call "Send.vi"("Message"=w298, "Queue Name"=w300) -> ()  [unwired: 9 in, 1 out]
          }
        }
        n130 = event-data("Discard?"=TRUE) -> ()  [unwired: 1 in, 1 out]
      }
      event Mouse Up {
        # "#NOTE\nAny changes here should be duplicated in the Mouse Up (Outside Pane) user event."
        # "Possible #BUG ?\nIf a left-mouse down is being simulated (via a right-click on a numeric), and then the right-mouse is released, a left-mouse up is simulated. LabVIEW then receives that left-mouse up and processes the command here.\n\nCould have a flag to indicate the left mouse up was simulated and ignore it?"
        n131 = event-data() -> ("Button"=w304:u16)  [unwired: 1 in, 7 out]
        n132 = case shown="1" w304 {
          tunnel: w303 -> [w305 w311 w315]
          tunnel: [w305 w311 cluster{"CtlRef":refnum<vi>, "Value":variant} {"CtlRef"=refnum, "Value"=variant}] -> w302
          frame Default {
          }
          frame 1 {
            # "#TODO\nPoll mouse buttons using Input Device Control for mouse up instead?"
            # "The Mouse Up event is sent to each deck to cancel a scratch.\n\nNote that the Mouse Up is for the entire pane (not just a jogwheel) as the mouse will more than likely NOT be over the jogwheel. This doesn't help the case where the mouse is released outside the window entirely."
            n133 = Bundle By Name(cluster=T9 {"Event"="", "Source"="", "Target"="", "Data"=variant} ("Message"), "Event"="Mouse Up" ("Type")) -> (w306:T9)
            n134 = call "Send.vi"("Message"=w306, "Queue Name"="Deck1") -> ()  [unwired: 9 in, 1 out]
            n135 = call "Send.vi"("Message"=w306, "Queue Name"="Deck2") -> ()  [unwired: 9 in, 1 out]
          }
          frame 2 {
            n136 = Unbundle(w315) -> ("CtlRef"=w313:refnum<vi>, "Value"=w312:variant)
            n137 = Not A Number/Path/Refnum?(number/path/refnum=w313) -> (NaN/Path/Refnum?=w314:bool)
            n138 = case shown="False" w314 {
              tunnel: w313 -> [w318 _]
              tunnel: w312 -> [w317 _]
              frame False {
                # "Send a left mouse up"
                # "Reset the value"
                n139 = property class="Ctl"(reference=w318, "Val(Sgnl)"=w317) -> ()  [unwired: 1 in, 2 out]
                n140 = dll-call lib="user32.dll" fn="SendInput"("nInputs"=u32 1, "pInputs"=T10 {"type"=0, "KEYBDINPUT"={"dx"=0, "dy"=0, "mouseData"=0, "dwFlags"=4, "time"=0, "dwExtraInfo"=0}} ("input"), "cbSize"=u32 28) -> ()  [unwired: 7 in, 2 out]
              }
              frame True {
              }
            }
          }
        }
      }
    }
  }
  n141 = Unregister For Events(event registration refnum=w29) -> ()  [unwired: 1 in, 1 out]
  n142 = Release Queue(queue=w18, force destroy? (F)=TRUE, error in (no error)=w25) -> ()  [unwired: 3 out]
